vi "DHE_DRV_set_roi.vi"(0 "fd":i32, 1 "xlenght":i32, 2 "ylenght":i32, 5 "xstart":i32, 7 "ystart":i32, 11 "error in (no error)":errorcluster) -> (4 "fd out":i32, 8 "return value":i32, 15 "error out":errorcluster)   [LabVIEW 2016]
doc: "This VI closes the I/O interface with the instrument."
uses:
  c/lib/libarcDHE.so
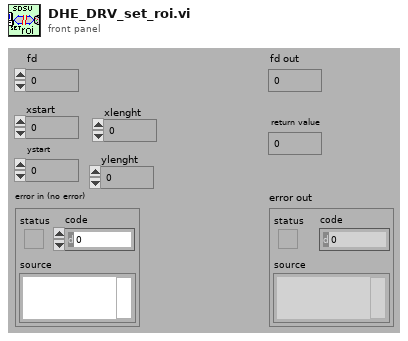
[diagram p1: front panel]
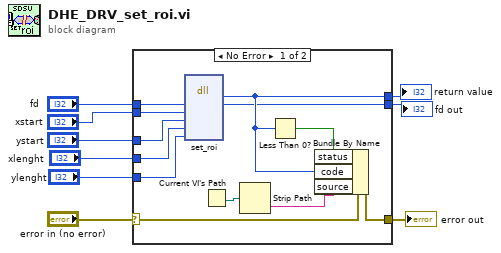
[diagram p0: block diagram]
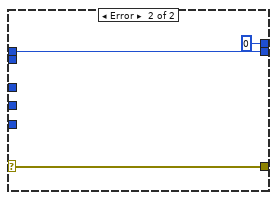
[diagram p2: hidden frame]
diagram:
  n1 = case shown="No Error" "error in (no error)" {
    selector: "error in (no error)" -> [w12 w22]
    tunnel: "fd" -> [w21 w24]
    tunnel: [w19 0] -> w8
    tunnel: [w16 w22] -> w7
    tunnel: "xstart" -> [w15 _]
    tunnel: "ystart" -> [w14 _]
    tunnel: [w13 w24] -> w4
    tunnel: "xlenght" -> [w11 _]
    tunnel: "ylenght" -> [w10 _]
    frame No Error {
      n2 = dll-call lib="home/simager/panview/PAN/Modules/SDSU/private/c/lib/libarcDHE.so" fn="set_roi"("fd"=w21, "xstart"=w15, "ystart"=w14, "xlen"=w11, "ylen"=w10) -> (w19:i32, "fd"=w13:i32)  [unwired: 7 in, 2 out]
      n3 = Current VI's Path() -> (path=w18:path)
      n4 = Strip Path(path=w18) -> (name=w17:string)  [unwired: 1 out]
      n5 = Less Than 0?(x=w19) -> (x < 0?=w20:bool)
      n6 = Bundle By Name(cluster=w12, "status"=w20, "code"=w19, "source"=w17) -> (w16:errorcluster)
    }
    frame Error {
    }
  }
  "error out" <- w7
  "return value" <- w8
  "fd out" <- w4
